vi "GetTable.vi"(7 "condition":string, 8 "error in (no error)":errorcluster, 9 "Primary":bool, 10 "table":string="#software", 11 "Database in":refnum<class "Database.lvclass">) -> (0 "error out":errorcluster, 1 "columns":string[](array[string]), 2 "data":string[][](array[string]), 3 "Database out":refnum<class "Database.lvclass">)   [LabVIEW 2016, in "Database.lvclass"]
uses:
  Database.lvclass
  Database.lvclass/Database.ctl
  <vilib>/addons/database/Connection.llb/Conn Execute.vi
  <vilib>/addons/database/Recordset.llb/Rec Fetch Recordset Data (R).vi
  <vilib>/addons/database/Recordset.llb/Rec Destroy - Connection.vi
  <vilib>/addons/database/_DB Variant To Data/Database Variant To Data.xnode
  <vilib>/addons/database/NI_Database_API.lvlib
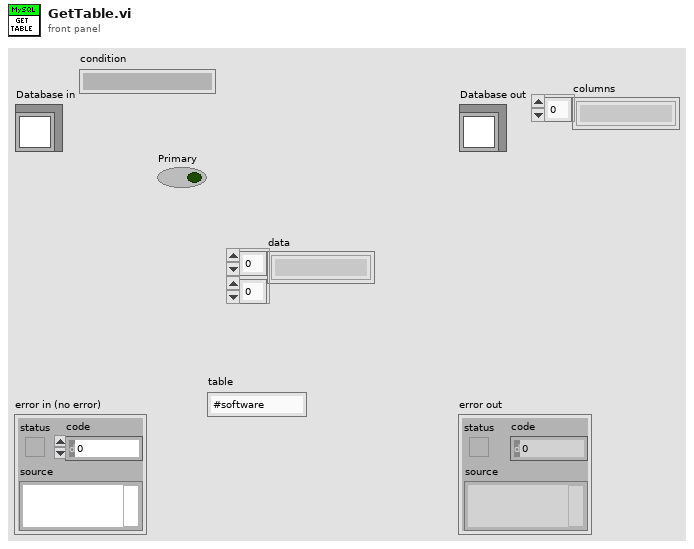
[diagram p1: front panel]
types:
  T1 = typedef "NI_Database_API.lvlib/Conn ObjectReference.ctl" = refnum<k1>
  T2 = typedef "NI_Database_API.lvlib/Rec ObjectReference.ctl" = refnum<k1>
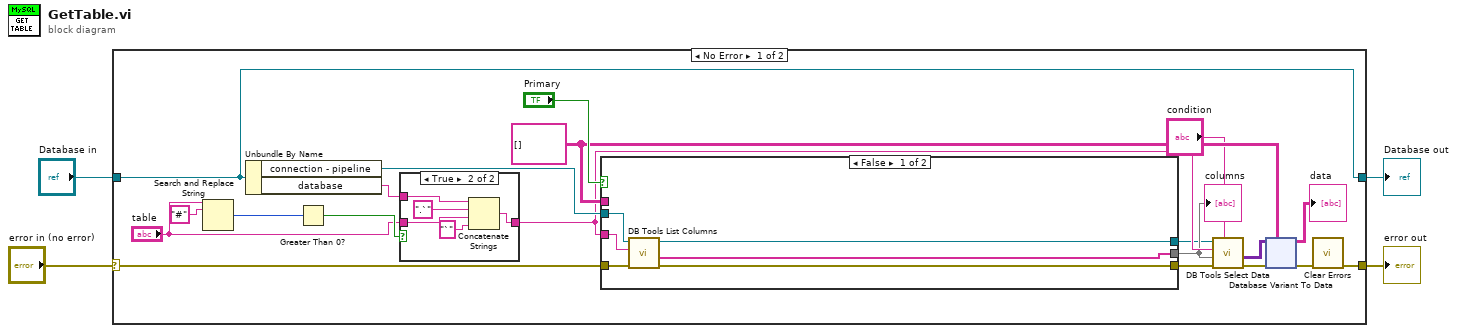
[diagram p0: block diagram]
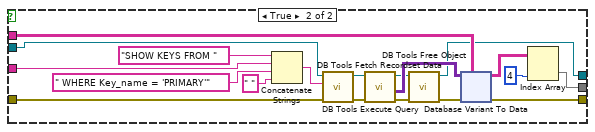
[diagram p2: hidden frame]
diagram:
  n1 = case shown="No Error" "error in (no error)" {
    selector: "error in (no error)" -> [w15 w145]
    tunnel: [w23 w145] -> w3
    tunnel: [w24 w144] -> w1
    tunnel: "Database in" -> [w24 w144]
    frame No Error {
      w10 = string[][] []
      n2 = Search and Replace String(input string="table", search string="#") -> (number of replacements=w21:i32)  [unwired: 6 in, 3 out]
      n3 = Unbundle By Name(w24) -> ("connection - pipeline"=w16:T1, "database"=w19:string)
      n4 = Greater Than 0?(x=w21) -> (x > 0?=w20:bool)
      n5 = case shown="True" w20 {
        tunnel: w19 -> [_ w142]
        tunnel: "table" -> [w138 w140]
        tunnel: [w138 w139] -> w8
        frame False {
        }
        frame True {
          n6 = Concatenate Strings(w142, ".`" ("string"), w140, "`" ("string")) -> (w139:string)
        }
      }
      n7 = case shown="False" "Primary" {
        tunnel: w8 -> [w72 w84]
        tunnel: w16 -> [w74 w82]
        tunnel: w15 -> [w73 w81]
        tunnel: [w70 w79] -> w12
        tunnel: w10 -> [_ w78]
        tunnel: [w71 w77] -> w7
        tunnel: [w69 w76] -> w6
        frame False {
          n8 = call <vilib>:"DB Tools List Columns.vi"("error in (no error)"=w73, "table"=w72, "connection reference"=w74) -> ("error out"=w70:errorcluster, "columns"=w71:string[], "connection reference out"=w69:T1)  [unwired: 1 in, 1 out]
        }
        frame True {
          n9 = Concatenate Strings("SHOW KEYS FROM ", w84, " WHERE Key_name = 'PRIMARY'", " " ("Substring")) -> (w83:string)
          n10 = call-poly <vilib>:"DB Tools Execute Query.vi"("error in (no error)"=w81, "SQL query"=w83, "connection reference"=w82) -> ("error out"=w90:errorcluster, "recordset reference"=w89:T2)  [unwired: 5 in]
          n11 = call-poly <vilib>:"DB Tools Fetch Recordset Data.vi"("error in (no error)"=w90, "recordset reference"=w89) -> ("error out"=w91:errorcluster, "recordset data"=w92:variant[][], "recordset reference out"=w88:T2)  [unwired: 3 in]
          n12 = call-poly <vilib>:"DB Tools Free Object.vi"("error in (no error)"=w91, "recordset reference"=w88) -> ("error out"=w80:errorcluster, "connection reference"=w76:T1)  [unwired: 8 in]
          n13 = xnode "Database Variant To Data"("database variant"=w92, "error in (no error)"=w80, "type"=w78) -> ("data"=w75:string[][], "error out"=w79:errorcluster)
          n14 = Index Array(array=w75, index (col)=4 ("disabled index (col)")) -> (element=w77:string[])  [unwired: 1 in]
        }
      }
      "columns" <- w7
      n15 = call <vilib>:"DB Tools Select Data.vi"("condition"="condition", "error in (no error)"=w12, "columns"=w7, "table"=w8, "connection reference"=w6) -> ("error out"=w13:errorcluster, "data"=w14:variant[][])  [unwired: 1 in, 1 out]
      n16 = xnode "Database Variant To Data"("database variant"=w14, "error in (no error)"=w13, "type"=w10) -> ("data"=→"data":string[][], "error out"=w11:errorcluster)
      n17 = call <vilib>:"Clear Errors.vi"("error in (no error)"=w11) -> ("error out"=w23:errorcluster)  [unwired: 5 in, 1 out]
    }
    frame Error {
    }
  }
  "error out" <- w3
  "Database out" <- w1
